vi "second_order_system.calculate.vi"(8 "sampling_time (s)":dbl, 9 "damping_ratio (zeta)":dbl=0.04, 10 "natural_freq (wn in Hz)":dbl=75.0, 11 "gain (K)":dbl=1.0) -> (2 "a1...an":dbl[](array[numeric]), 3 "b0...bn":dbl[](array[numeric]))   [LabVIEW 2015, in "discrete_control_systems.lvlib"]
doc: "Calculates the gains for a second order transfer function in the continous domain to be used for a discrete domain difference equation. The calculation usese the provided Gain (K), Natural Frequency (wn), and Damping Ratio (zeta) paramenters and the sampling time. For this calculation we place two zeros at z = -1 + j0.\n\nThe continous transfer function has the following equation in the LaPlace domain, where Y(s) is the transfer function output given a U(s) intput:\n\nY(s) K * wn^2\n---- = ----------------------------\nU(s) s^2 + 2*zeta*wn + wn^2 \n\nThe sampling_time input represents how fast will the control loop run and is necessary in order to allow for an accurate implementation of the controller with parameters that can be reused for multiple sampling times."
uses:
  discrete_control_systems.lvlib
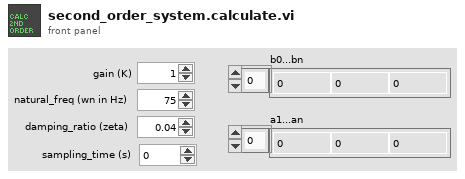
[diagram p1: front panel]
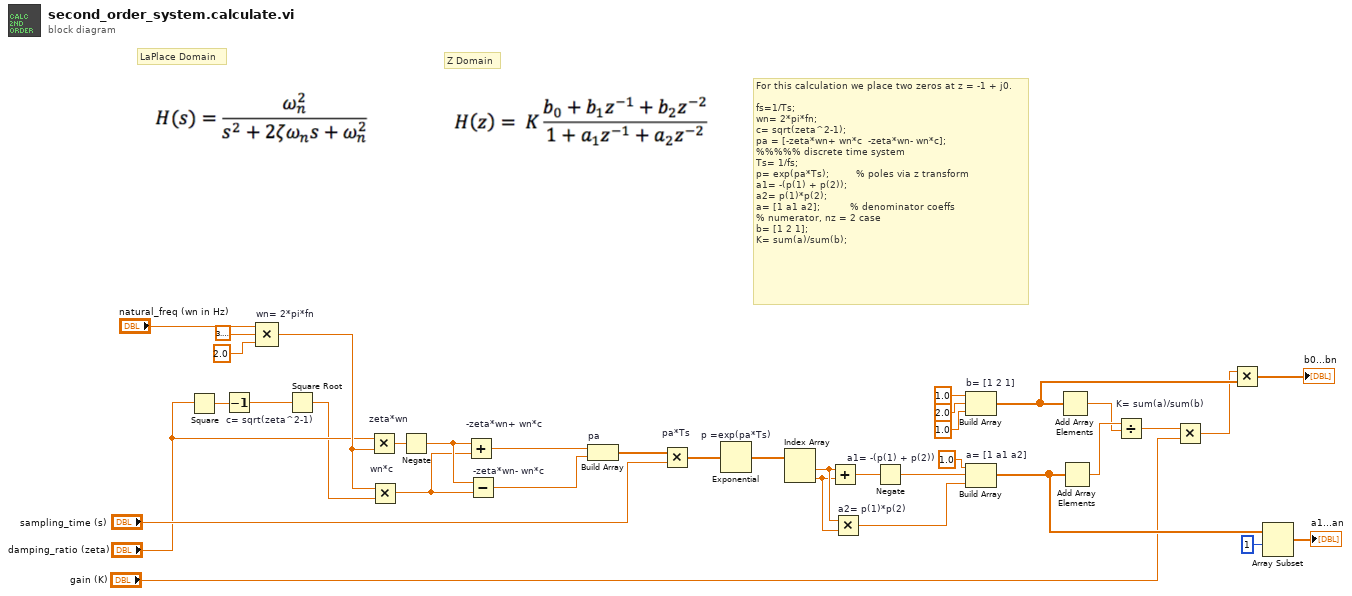
[diagram p0: block diagram]
diagram:
  # "Z Domain"
  # "LaPlace Domain"
  # "For this calculation we place two zeros at z = -1 + j0.\n\nfs=1/Ts;\nwn= 2*pi*fn;\nc= sqrt(zeta^2-1);\npa = [-zeta*wn+ wn*c  -zeta*wn- wn*c];\n%%%%% discrete time system\nTs= 1/fs;\np= exp(pa*Ts);         % poles via z transform\na1= -(p(1) + p(2));\na2= p(1)*p(2);\na= [1 a1 a2];          % denominator coeffs\n% numerator, nz = 2 case\nb= [1 2 1];\nK= sum(a)/sum(b);"
  n1 = Square(x="damping_ratio (zeta)") -> (x^2=w35:dbl)
  n2 = Decrement(x=w35) -> (x-1=w34:cdb)
  n3 = Compound Arithmetic op=MULTIPLY "wn= 2*pi*fn"("natural_freq (wn in Hz)", 3.141592653589793, 2.0 ("value")) -> (w19:dbl)
  n4 = Square Root "c= sqrt(zeta^2-1)"(x=w34) -> (sqrt(x)=w13:cdb)
  n5 = Multiply "zeta*wn"(x="damping_ratio (zeta)", y=w19) -> (x*y=w15:dbl)
  n6 = Multiply "wn*c"(x=w19, y=w13) -> (x*y=w14:cdb)
  n7 = Negate(x=w15) -> (-x=w16:dbl)
  n8 = Add "-zeta*wn+ wn*c"(x=w16, y=w14) -> (x+y=w33:cdb)
  n9 = Subtract "-zeta*wn- wn*c"(x=w16, y=w14) -> (x-y=w32:cdb)
  n10 = Build Array "pa"(w33, w32) -> (w31:cdb[])
  n11 = Multiply "pa*Ts"(x=w31, y="sampling_time (s)") -> (x*y=w30:cdb[])
  n12 = Exponential "p =exp(pa*Ts)"(1:w30) -> (0:w29:cdb[])
  n13 = Index Array(array=w29) -> (element #1=w27:cdb, element #2=w26:cdb)  [unwired: 2 in]
  n14 = Add(x=w27, y=w26) -> (x+y=w28:cdb)
  n15 = Multiply "a2= p(1)*p(2)"(x=w27, y=w26) -> (x*y=w23:cdb)
  n16 = Negate "a1= -(p(1) + p(2))"(x=w28) -> (-x=w24:cdb)
  n17 = Build Array "b= [1 2 1]"(1.0 ("element"), 2.0 ("element"), 1.0 ("element")) -> (w5:dbl[])
  n18 = Build Array "a= [1 a1 a2]"(1.0 ("element"), w24, w23) -> (w7:cdb[])
  n19 = Add Array Elements(numeric array=w5) -> (sum=w9:dbl)
  n20 = Add Array Elements(numeric array=w7) -> (sum=w10:cdb)
  n21 = Divide "K= sum(a)/sum(b)"(x=w10, y=w9) -> (x/y=w2:cdb)
  n22 = Multiply(x=w2, y="gain (K)") -> (x*y=w1:cdb)
  n23 = Multiply(x=w1, y=w5) -> (x*y=→"b0...bn":cdb[])
  n24 = Array Subset(array=w7, index=1) -> (→"a1...an":cdb[])  [unwired: 1 in]
